vi "Main.vi"() -> ()   [LabVIEW 2016]
uses:
  Spreadsheet filling/Controls/Language Control.ctl
  <vilib>/Platform/TimedLoop/XDataNode/timing_clust.ctl
  <vilib>/Platform/TimedLoop/XDataNode/nitl_modes.ctl
  <vilib>/Platform/TimedLoop/XDataNode/wakeup.ctl
  types/final data type.ctl
  <vilib>/Utility/config.llb/Read Key (Boolean).vi
  <vilib>/Platform/TimedLoop/XDataNode/XDataNode.xnode
  <vilib>/Platform/TimedLoop/XDataNode/XDNodeRunTimeDep.lvlib
  <vilib>/Utility/config.llb/NI_LVConfig.lvlib
panel:
  in  "Gas":bool
  out "Volume % Difference":dbl
  out "Progress":dbl(slide) scale=0.0..100.0
  in  "Software Version":string="1.09(US)"
  out "Sample in progress":bool
  out "Collect info done":bool
  in  "Sample method 2":u16(ring) items=["None", "Pulse Input", "Current Input", "Serial Input"]
  out "Mass % Difference":dbl
  in  "Sample \ninterval (S)":dbl=30.0
  in  "Language":T1
  in  "Collect info":bool
  in  "Export report":bool
  in  "Reset table":bool
  in  "Setpoint \n(kg/min)":dbl
  out "Data table":string[][](table)
  in  "Sample method 1":u16(ring) items=["None", "Pulse Input", "Current Input", "Serial Input"]
  in  "Begin pulse sample":bool
  in  "Transfer Data":bool
  in  "Run #":u16
  # "Mass\n(UUT)"
  # "Mass\n(Master)"
  # "Mass \n% diff"
  # "Volume\n(UUT)"
  # "Volume\n(Master)"
  # "Setpoint"
  # "Run"
  # "Select an input type"
  # "Select an input type"
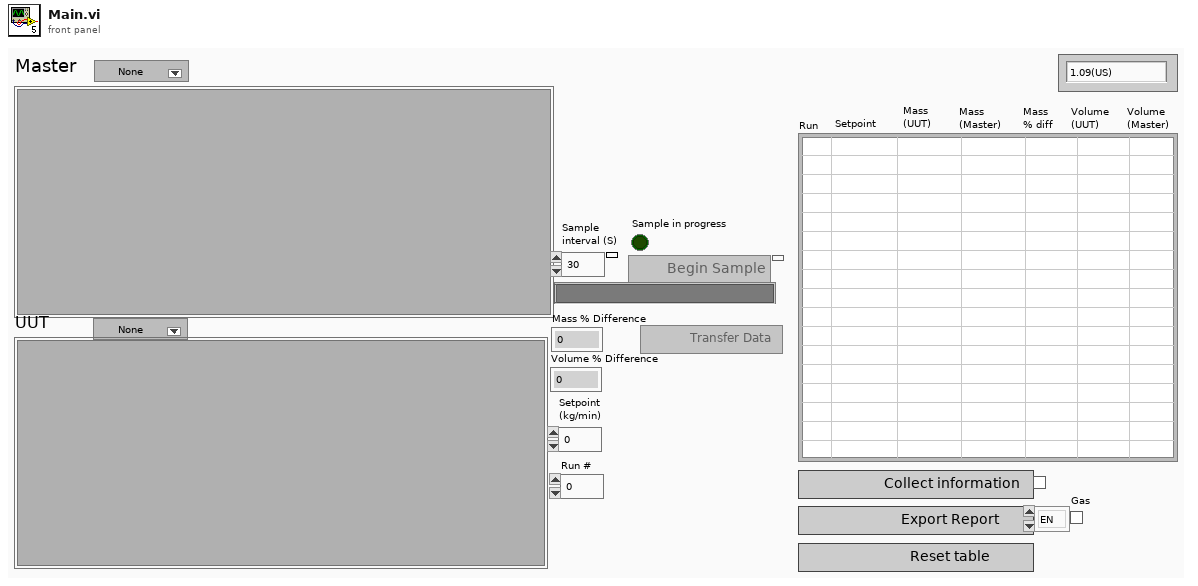
[diagram p1: front panel]
types:
  T1 = typedef "Language Control.ctl" = enum16{"EN", "ES", "FR", "RU"}
  T2 = typedef "final data type.ctl" = cluster{"Master final data":cluster{"Mass total":dbl, "Volume total":dbl, "Density mean":dbl}, "UUT final data":cluster{"Mass total":dbl, "Volume total":dbl, "Density mean":dbl}}
  T3 = enum16{"Init", "Transfer data", "Sample started", "Sample complete"}
  T4 = typedef "XDNodeRunTimeDep.lvlib/timing_clust.ctl" = cluster{"Expected End [f-1]":u64, "Actual End [f-1]":u64, "Finished Late? [f-1]":bool, "Expected End [i-1]":u64, "Actual End [i-1]":u64, "Finished Late? [i-1]":bool, "Expected Start [i]":u64, "Actual Start [i]":u64, "Expected Start [f]":u64, "Actual Start [f]":u64, "Source Name":string, "Structure Name":string, "Period":i64, "Deadline":i64, "Offset":i64, "Start":i64, "Priority":i32, "Timeout":i32, "Mode":T5, "Wakeup Reason":T6, "Error":errorcluster, "Source Type":string, "Secondary Source Type":string, "Global End Time":u64, "Global Start Time":u64, "Frame Duration":u64, "Iteration Duration":u64, "Assigned CPU":i32, "I/O Scan Engine Mode":u32}
  T5 = typedef "XDNodeRunTimeDep.lvlib/nitl_modes.ctl" = enum32{"No Change", "Process missed periods, maintain original phase", "Discard missed periods, maintain original phase", "Process missed periods, ignore original phase", "Discard missed periods, ignore original phase"}
  T6 = typedef "XDNodeRunTimeDep.lvlib/wakeup.ctl" = enum32{"Normal", "Aborted", "Asynchronous wakeup", "Timing source error", "Timed loop error", "Timeout"}
  T7 = enum8{"Enabled", "Disabled", "Disabled and Grayed Out"}
  T8 = typedef "NI_LVConfig.lvlib/Config Data RefNum.ctl" = refnum<k1>
  T9 = typedef "Information_tab_type.ctl" = cluster{"Test Date and Time, 1":string, "Test Comments,3":string, "Sensor Serial Number,6":string, "Sensor Model,7":string, "Size,8":string, "Material,9":string, "Press rating, 10":string, "Temp rating, 11":string, "FCF, 14":string, "D1, 15":string, "D2, 16":string, "K1, 17":string, "K2, 18":string, "FD, 19":string, "Density Temp Coeff, 20":string, "Transmitter Serial Number,23":string, "Transmitter Model Number,24":string, "Mass Flow Units, 25":string, "Density Units, 26":string, "Temperature Units, 27":string, "Mass Flow Cutoff, 28":string, "Mass Flow Damping, 29":string, "Flow Direction, 30":string, "Frequency Flow Rate, 31":string, "Frequency Span, 32":string, "Flow Accuracy, 35":string, "Flow Repeatability, 36":string, "Zero Stability, 37":string, "Density Accuracy, 38":string, "Density Repeatability, 39":string, "Nomincal Flow Rate, 41":string, "Meter Zero, 43":string, "Status, 45":string, "Customer name, 46":string, "Customer address, 47":string, "Sales order number, 48":string, "Technician Name, 49":string, "ref meter, 50":string, "product code,51":string, "fluid,52":string, "fluid temp,53":string}
  T10 = enum16{"0-1-2-3", "2-3-0-1", "1-0-3-2", "3-2-1-0"}
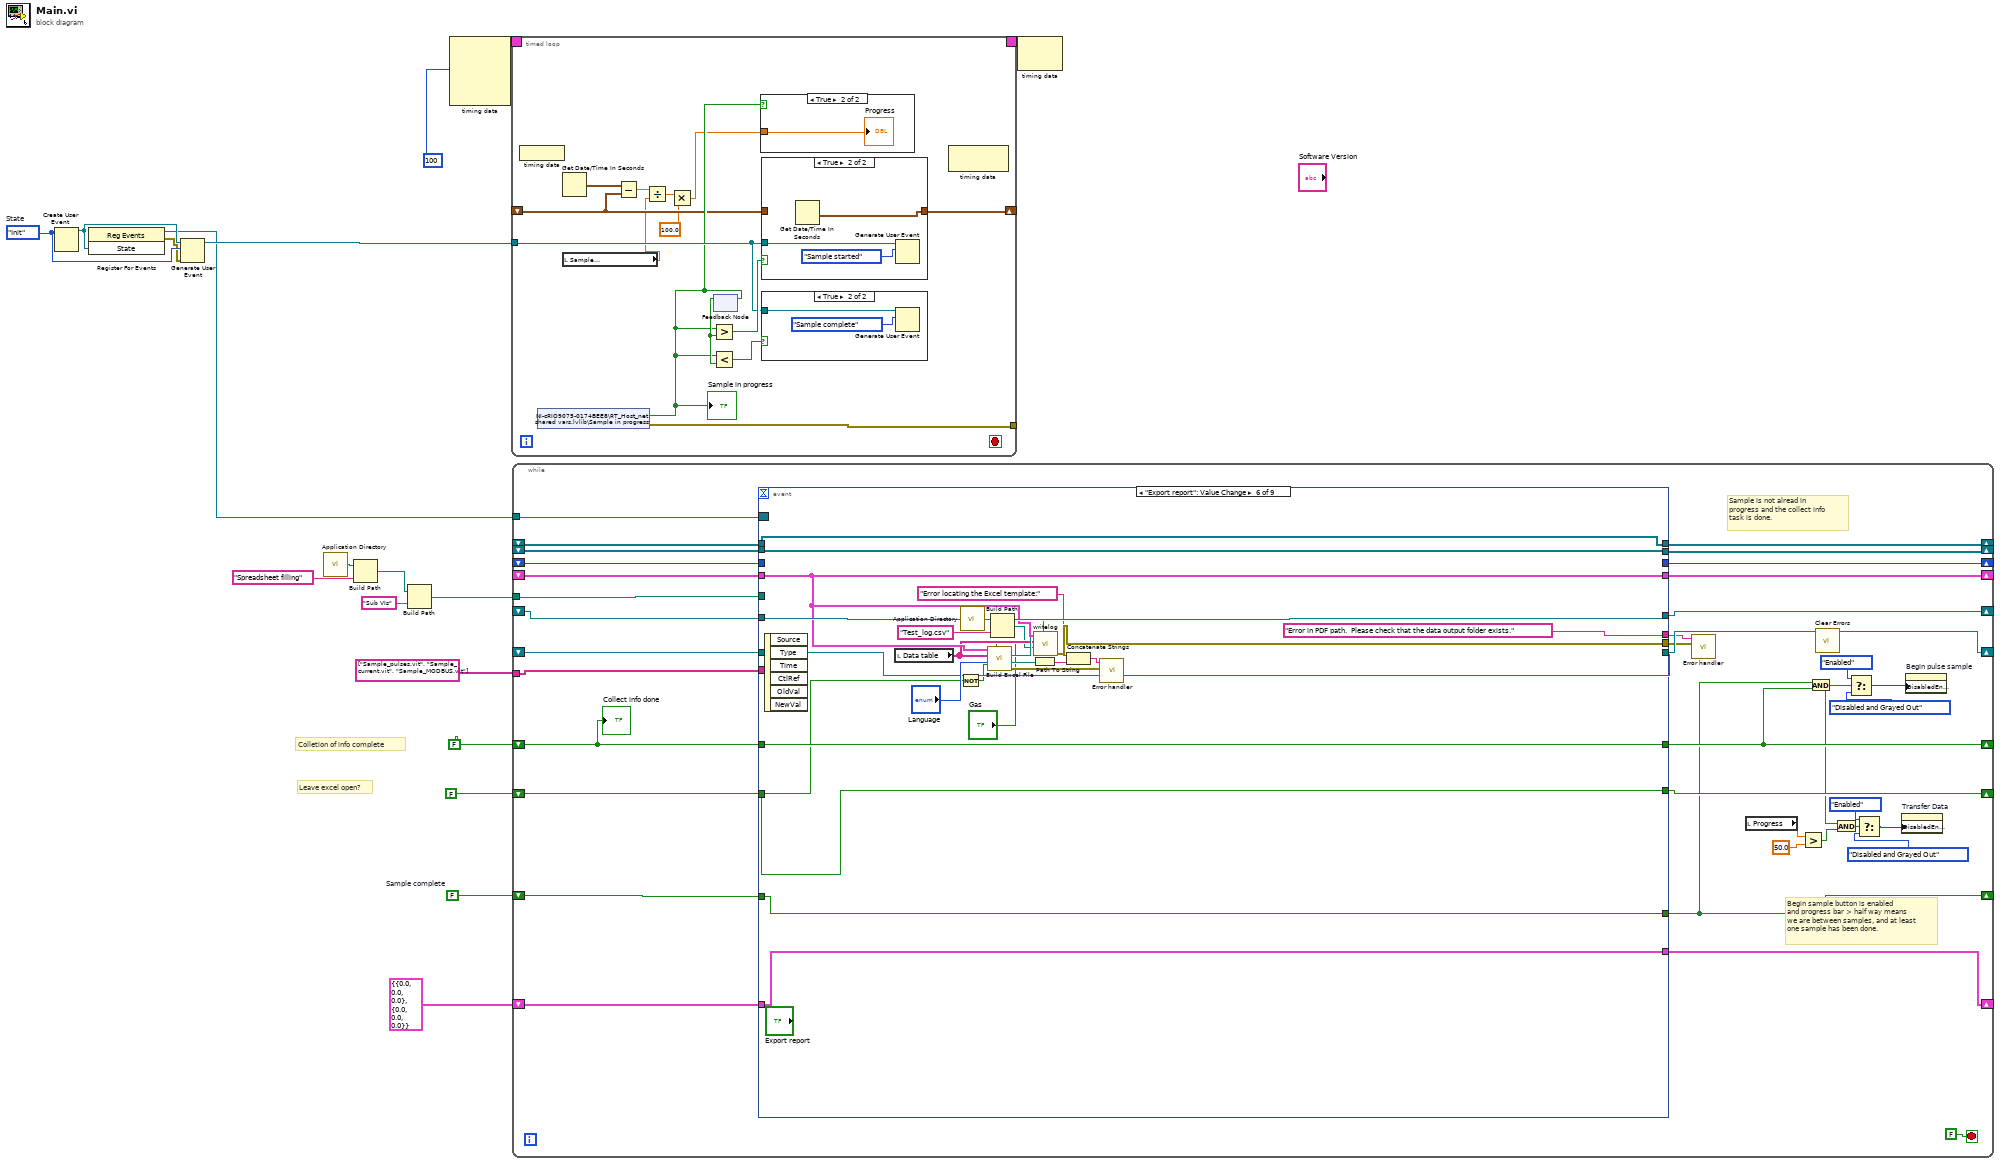
[diagram p0: block diagram]
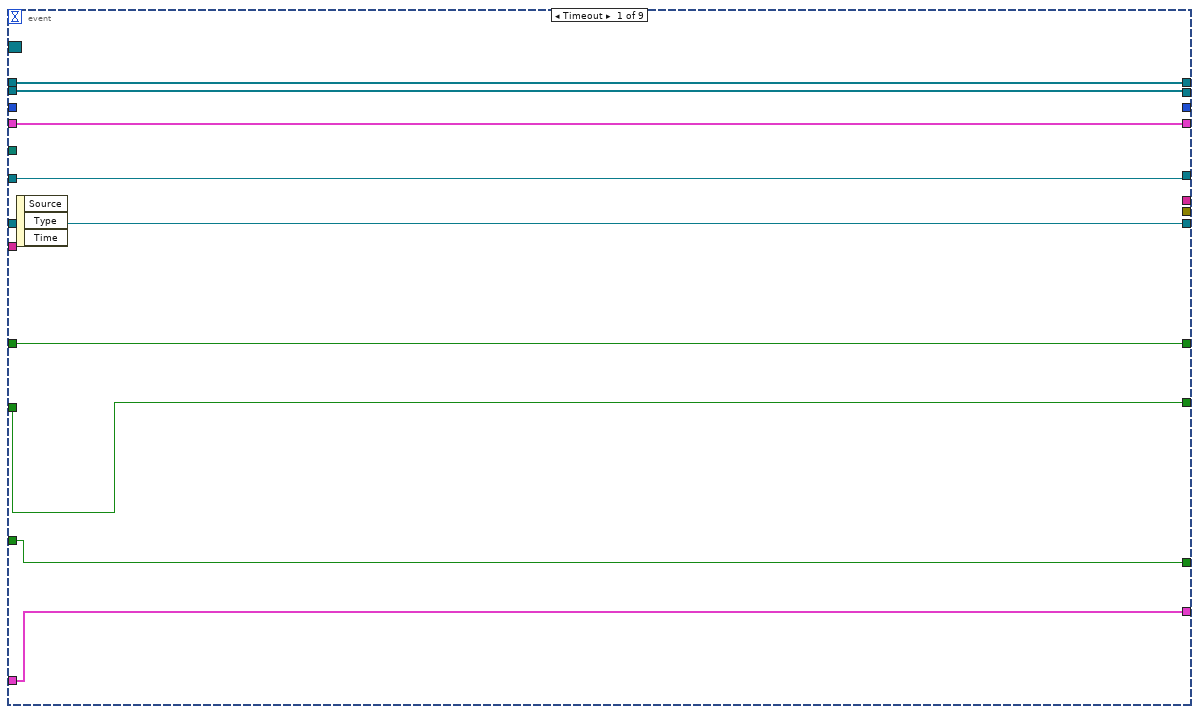
[diagram p5: hidden frame]
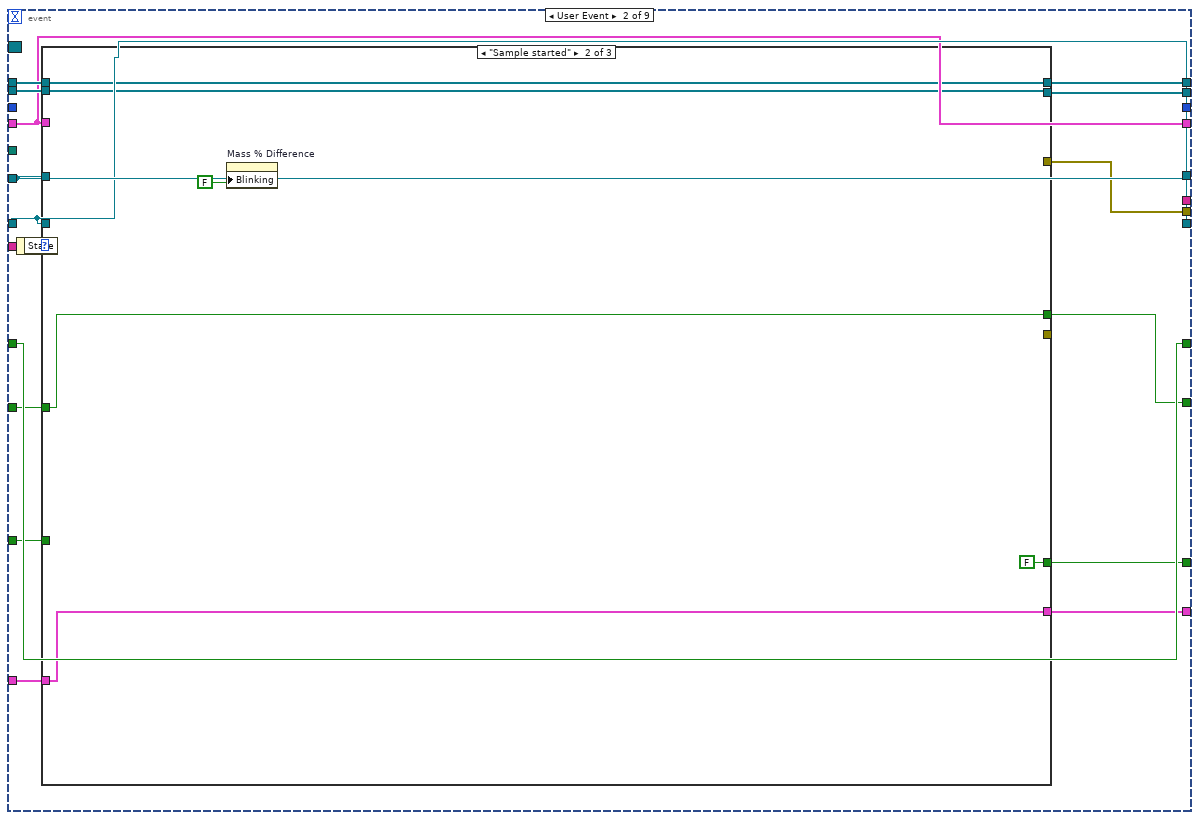
[diagram p6: hidden frame]
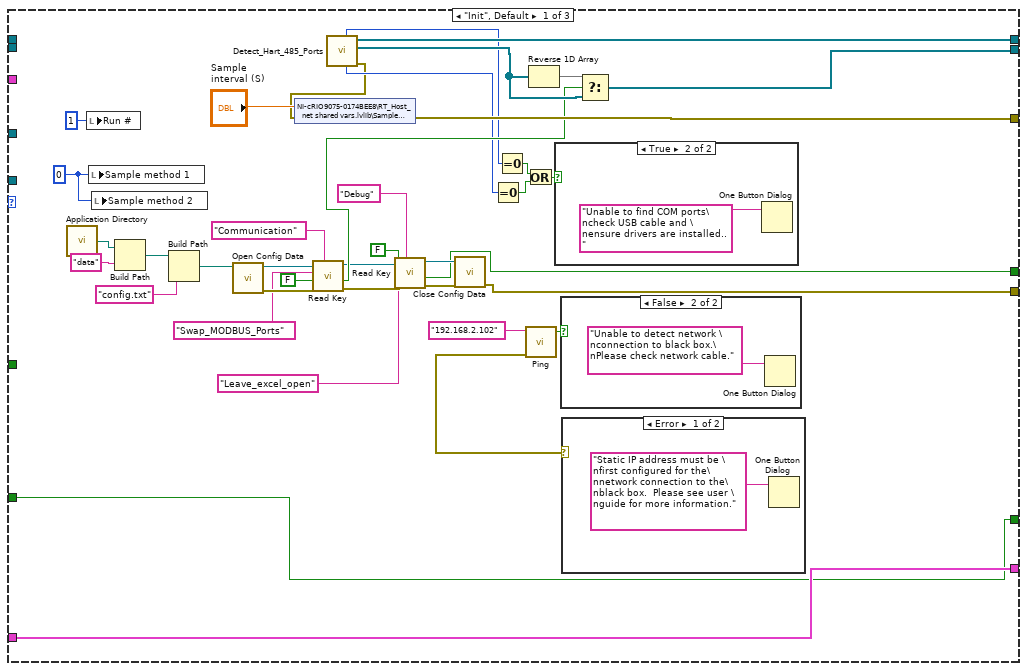
[diagram p7: hidden frame]
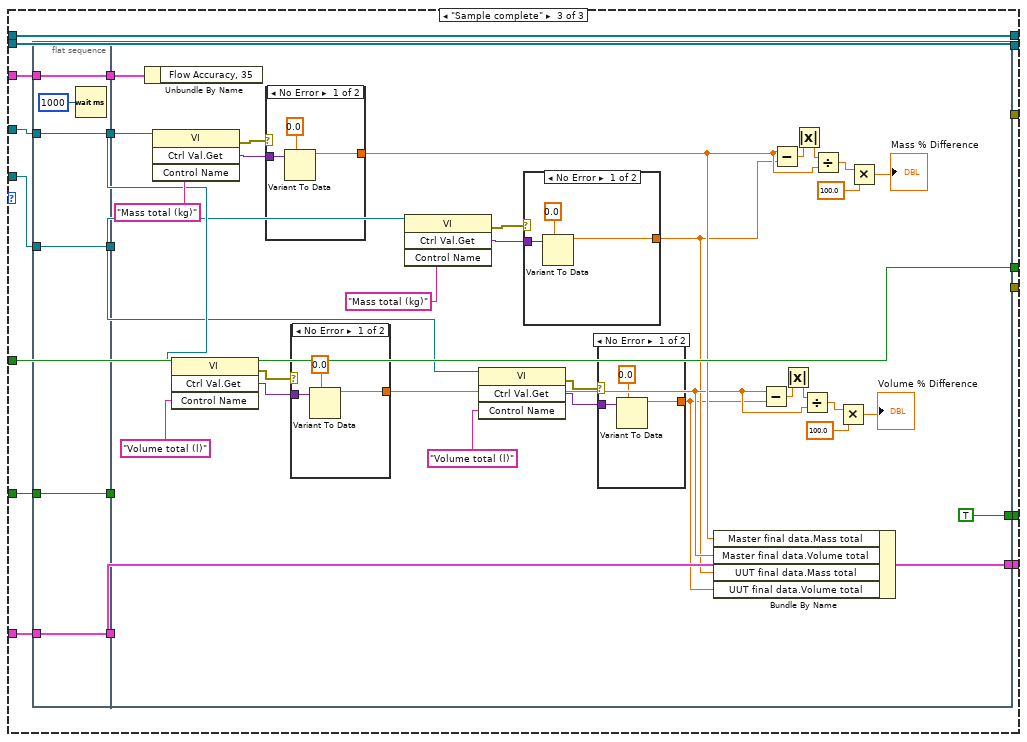
[diagram p11: hidden frame]
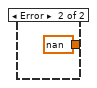
[diagram p12: hidden frame]
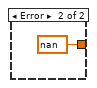
[diagram p13: hidden frame]
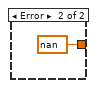
[diagram p14: hidden frame]
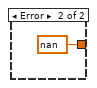
[diagram p15: hidden frame]
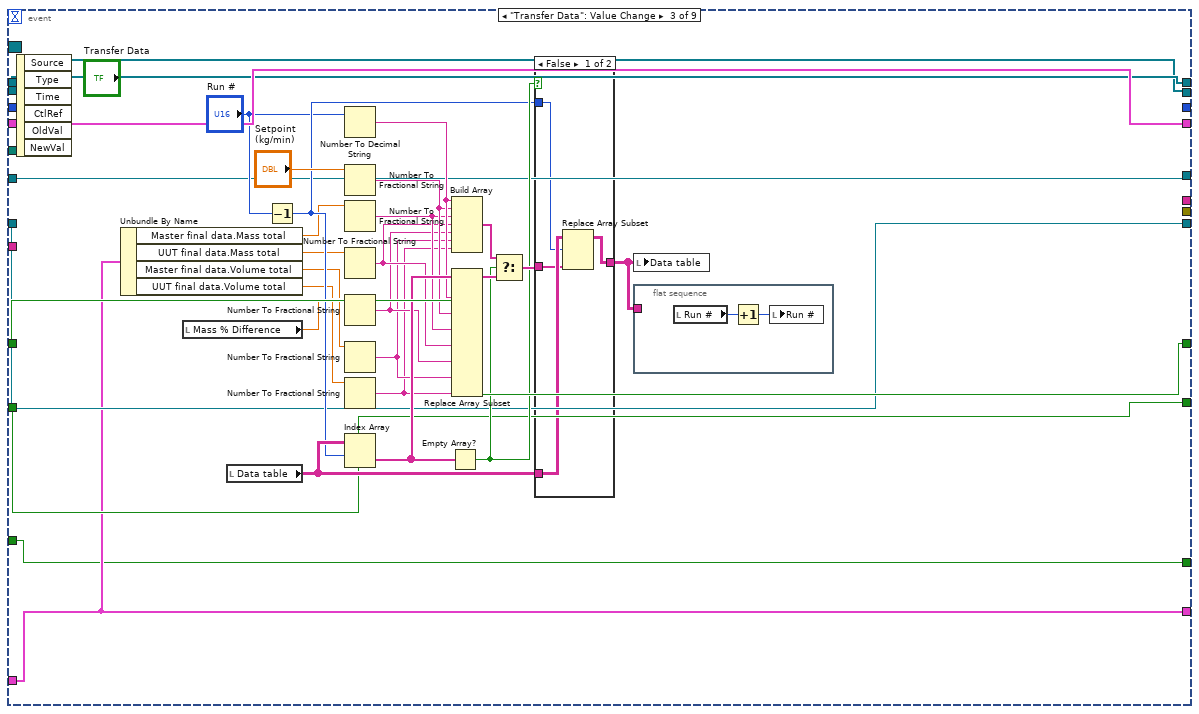
[diagram p16: hidden frame]
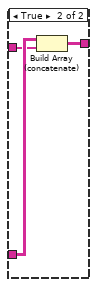
[diagram p17: hidden frame]
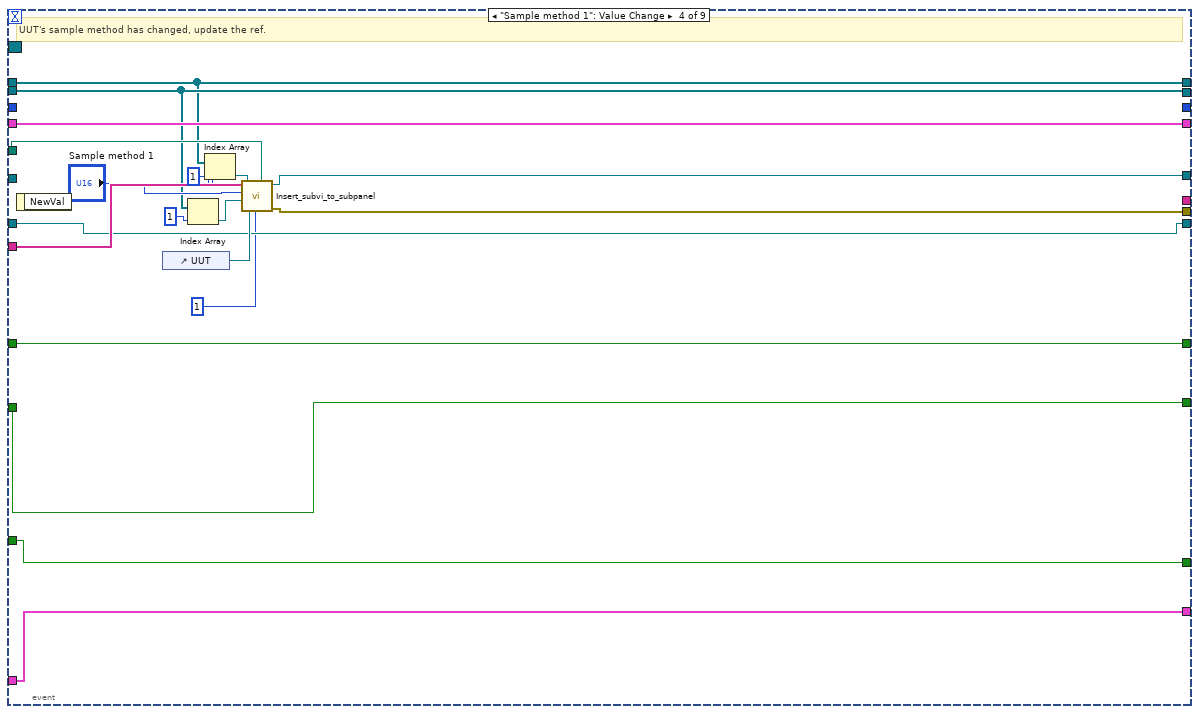
[diagram p18: hidden frame]
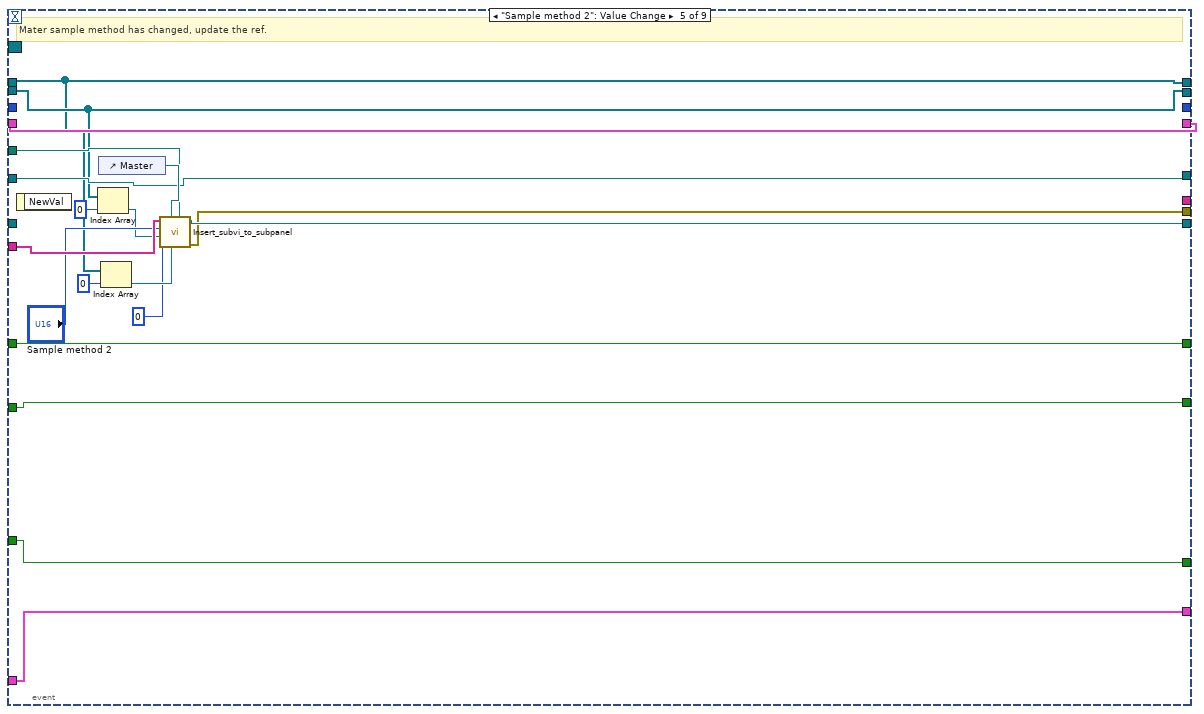
[diagram p19: hidden frame]
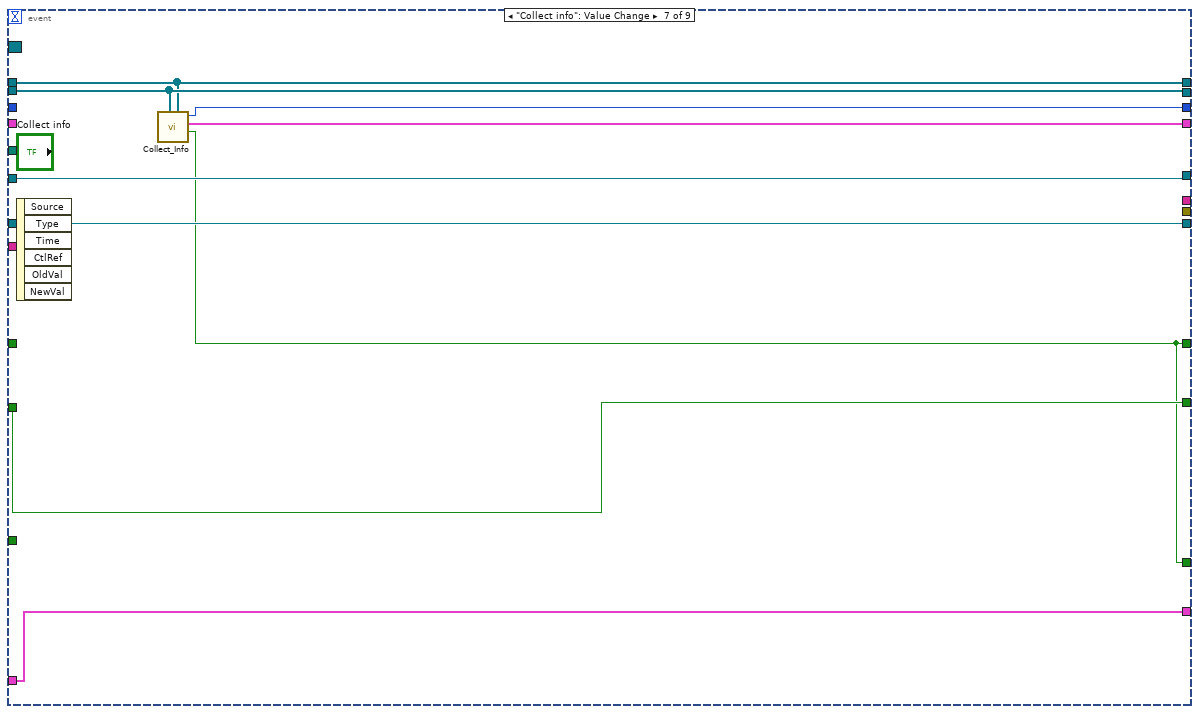
[diagram p20: hidden frame]
diagram:
  w1 = FALSE  # Sample complete
  w12 = T3."Init"  # State
  # "Leave excel open?"
  # "Colletion of info complete"
  n1 = Create User Event(user event datatype=w12) -> (user event=w11:refnum<user-event>)  [unwired: 1 in, 1 out]
  n2 = register-events(w11) -> (reference out=w4:refnum<event-registration>, error out=w10:errorcluster)  [unwired: 2 in]
  n3 = Generate User Event(user event=w11, event data cluster=w12, error in=w10) -> (user event out=w5:refnum<user-event>)  [unwired: 1 in, 1 out]
  n4 = call <vilib>:"Application Directory.vi"() -> ("Application Directory"=w18:path)
  n5 = Build Path(base path=w18, name or relative path="Spreadsheet filling") -> (appended path=w16:path)
  n6 = Build Path(base path=w16, name or relative path="Sub VIs") -> (appended path=w14:path)
  n7 = node-c288(i64 100 ("Period")) -> (w8:T4)  [unwired: 3 in]
  n8 = timed-loop {
    timing: w8 -> [_]
    timing-out: [_] -> w7
    tunnel: [w32] -> _
    tunnel: w5 -> [w29]
    shift-right: [w26] -> _
    shift-left: _ -> [w24]
    stop <- _ stop-if-true
    n9 = node-c288() -> ()  [unwired: 1 in]
    n10 = shared-variable "NI-cRIO9075-0174BEE8\\RT_Host_net shared vars.lvlib\\Sample in progress"() -> (w27:bool, error out=w32:errorcluster)  [unwired: 1 in]
    "Sample in progress" <- w27
    n11 = local read "Sample \ninterval (S)"() -> (w22:dbl)
    n12 = Get Date/Time In Seconds() -> (seconds since 1Jan1904=w25:timestamp)
    n13 = Subtract(x=w25, y=w24) -> (x-y=w23:dbl)
    n14 = Divide(x=w23, y=w22) -> (x/y=w21:dbl)
    n15 = Multiply(x=w21, y=100.0) -> (x*y=w19:dbl)
    n16 = feedback-in #1(w27) -> ()
    n17 = feedback #1() -> (w30:bool)  [unwired: 1 in]
    n18 = Greater?(x=w27, y=w30) -> (0:w31:bool)
    n19 = Less?(x=w27, y=w30) -> (x < y?=w28:bool)
    n20 = case shown="True" w27 {
      tunnel: w19 -> [_ w33]
      frame False {
      }
      frame True {
        "Progress" <- w33
      }
    }
    n21 = case shown="True" w31 {
      tunnel: w29 -> [_ w39]
      tunnel: [w36 w37] -> w26
      tunnel: w24 -> [w36 _]
      frame False {
      }
      frame True {
        n22 = Get Date/Time In Seconds() -> (seconds since 1Jan1904=w37:timestamp)
        n23 = Generate User Event(user event=w39, event data cluster=T3."Sample started" ("event data")) -> ()  [unwired: 2 in, 2 out]
      }
    }
    n24 = case shown="True" w28 {
      tunnel: w29 -> [_ w35]
      frame False {
      }
      frame True {
        n25 = Generate User Event(user event=w35, event data cluster=T3."Sample complete" ("event data")) -> ()  [unwired: 2 in, 2 out]
      }
    }
    n26 = node-c288() -> ()  [unwired: 1 in, 1 out]
  }
  n27 = while {
    shift-right: [w77] -> _
    shift-left: _ -> [w74]
    tunnel: string[] ["Sample_pulses.vit", "Sample_current.vit", "Sample_MODBUS.vit"] -> [w76]
    tunnel: w14 -> [w75]
    shift-right: [w73] -> _
    shift-left: _ -> [w72]
    tunnel: w4 -> [w71]
    shift-right: [w45] -> _
    shift-left: FALSE ("Collect info done") -> [w70]
    shift-right: [w69] -> _
    shift-left: _ -> [w68]
    shift-right: [w64] -> _
    shift-left: _ -> [w62]
    shift-right: [w63] -> _
    shift-left: _ -> [w61]
    shift-right: [w59] -> _
    shift-left: FALSE ("Collect info done") -> [w60]
    shift-right: [w56] -> _
    shift-left: _ -> [w55]
    shift-right: [w53] -> _
    shift-left: T2 {"Master final data"={"Mass total"=0.0, "Volume total"=0.0, "Density mean"=0.0}, "UUT final data"={"Mass total"=0.0, "Volume total"=0.0, "Density mean"=0.0}} ("Final data") -> [w54]
    shift-right: [w42] -> _
    shift-left: w1 -> [w43]
    stop <- FALSE stop-if-true
    # "Sample is not alread in\nprogress and the collect info \ntask is done."
    # "Begin sample button is enabled\nand progress bar > half way means \nwe are between samples, and at least\none sample has been done."
    n28 = event shown="[5] \"Export report\": Value Change" {
      selector: w71 -> [_ _ _ _ _ _ _ _ _]
      dyn-events: _ -> [_ _ _ _ _ _ _ _ _]
      timeout: _ -> [_ _ _ _ _ _ _ _ _]
      tunnel: w76 -> [_ _ _ w279 w296 _ _ _ _]
      tunnel: w75 -> [_ _ _ w271 w290 _ _ _ _]
      tunnel: [w87 w102 w227 w274 w293 w322 w331 w343 w356] -> w77
      tunnel: w74 -> [w87 w102 w227 _ w293 w322 w331 w343 w356]
      tunnel: [w86 w92 w251 w275 w292 w315 w330 w342 w355] -> w73
      tunnel: w72 -> [w86 w92 w251 w275 w292 w315 _ w342 w355]
      tunnel: w70 -> [w85 w101 w250 w272 w298 w320 _ _ w354]
      tunnel: [w85 w101 w250 w272 w298 w320 w323 w341 w354] -> w45
      tunnel: [_ w100 _ w276 w291 w316 _ _ _] -> w58
      tunnel: [w84 w99 w228 w273 w294 w319 w329 w340 w353] -> w69
      tunnel: w68 -> [w84 w99 w228 w273 _ w319 w329 w340 w353]
      tunnel: [w83 w98 w239 w267 w287 w318 w327 w339 w352] -> w64
      tunnel: [w82 w97 w238 w269 w289 w317 w328 w338 w351] -> w63
      tunnel: w62 -> [w83 w96 w239 w267 w287 w318 w327 w339 w352]
      tunnel: w61 -> [w82 w95 w238 w269 w289 w317 w328 w338 w351]
      tunnel: [w81 w94 w233 w263 w284 w309 w326 w333 w350] -> w59
      tunnel: w60 -> [w81 w93 w233 w263 w284 w309 w326 w333 w350]
      tunnel: [_ _ _ _ _ "Error in PDF path.  Please check that the data output folder exists." ("Error reason") _ _ _] -> w57
      tunnel: [_ _ _ _ _ _ w325 _ _] -> w56
      tunnel: w55 -> [_ _ _ _ _ _ _ _ _]
      tunnel: w54 -> [w80 w91 w222 w262 w281 w301 w324 w337 w349]
      tunnel: [w80 w90 w222 w262 w281 w301 w324 w337 w349] -> w53
      tunnel: w43 -> [w79 w89 w221 w261 w280 w300 _ w332 w348]
      tunnel: [w79 w88 w221 w261 w280 w300 w323 w332 w348] -> w42
      event Timeout {
        n29 = event-data() -> ()  [unwired: 1 in, 3 out]
      }
      event User Event {
        n30 = event-data() -> ("State"=w103:T3)  [unwired: 1 in]
        n31 = case shown="\"Sample started\"" w103 {
          tunnel: w102 -> [_ _ w166]
          tunnel: [w140 _ _] -> w100
          tunnel: w99 -> [_ _ w165]
          tunnel: [w139 w151 w164] -> w98
          tunnel: [w125 w150 w163] -> w97
          tunnel: w96 -> [_ w151 w164]
          tunnel: w95 -> [_ w150 w163]
          tunnel: [w107 _ _] -> _
          tunnel: [w106 w149 w160] -> w94
          tunnel: w93 -> [_ w149 w160]
          tunnel: w92 -> [_ _ w158]
          tunnel: w91 -> [w105 w147 w156]
          tunnel: [w105 w147 w155] -> w90
          tunnel: w89 -> [w104 _ w153]
          tunnel: [w104 FALSE ("Sample complete") w152] -> w88
          frame "Init", Default {
            w142 = u16 0 ("Run")
            n32 = call <vilib>:"Application Directory.vi"() -> ("Application Directory"=w136:path)
            n33 = local write "Run #"(u16 1 ("Run #")) -> ()
            n34 = local write "Sample method 1"(w142) -> ()
            n35 = local write "Sample method 2"(w142) -> ()
            n36 = Build Path(base path=w136, name or relative path="data") -> (appended path=w135:path)
            n37 = Build Path(base path=w135, name or relative path="config.txt") -> (appended path=w138:path)
            n38 = call <vilib>:"Open Config Data.vi"("configuration file path"=w138) -> ("error out"=w132:errorcluster, "refnum"=w133:T8)  [unwired: 8 in, 1 out]
            n39 = call-poly <vilib>:"Read Key.vi"("section"="Communication", "error in (no error)"=w132, "default value"=FALSE, "key"="Swap_MODBUS_Ports", "refnum"=w133) -> ("error out"=w113:errorcluster, "value"=w126:bool, "refnum out"=w114:T8)  [unwired: 3 in, 1 out]
            n40 = call "Detect_Hart_485_Ports.vi"() -> ("error out"=w118:errorcluster, "485 Ports"=w128:refnum<visa-resource-name>[], "HART ports"=w139:refnum<visa-resource-name>[], "# 485 ports found"=w124:i32, "# HART ports found"=w123:i32)  [unwired: 6 in, 1 out]
            n41 = shared-variable "NI-cRIO9075-0174BEE8\\RT_Host_net shared vars.lvlib\\Sample period"("Sample \ninterval (S)", error in=w118) -> (error out=w140:errorcluster)
            n42 = call-poly <vilib>:"Read Key.vi"("section"="Debug", "error in (no error)"=w113, "default value"=FALSE, "key"="Leave_excel_open", "refnum"=w114) -> ("error out"=w112:errorcluster, "value"=w106:bool, "refnum out"=w111:T8)  [unwired: 3 in, 1 out]
            n43 = call <vilib>:"Close Config Data.vi"("error in (no error)"=w112, "refnum"=w111) -> ("error out"=w107:errorcluster)  [unwired: 8 in, 1 out]
            n44 = Equal To 0?(x=w124) -> (x = 0?=w121:bool)
            n45 = Equal To 0?(x=w123) -> (x = 0?=w122:bool)
            n46 = Or(x=w122, y=w121) -> (x .or. y?=w120:bool)
            n47 = call "Ping.vi"("Host IP Address"="192.168.2.102") -> ("error out"=w115:errorcluster, "success"=w116:bool)  [unwired: 8 in, 1 out]
            n48 = Reverse 1D Array(array=w128) -> (reversed array=w127:refnum<visa-resource-name>[])
            n49 = case shown="True" w120 {
              frame False {
              }
              frame True {
                n50 = One Button Dialog(message="Unable to find COM ports\ncheck USB cable and \nensure drivers are installed..") -> ()  [unwired: 1 in, 1 out]
              }
            }
            n51 = case shown="False" w116 {
              frame True {
              }
              frame False {
                n52 = One Button Dialog(message="Unable to detect network \nconnection to black box.\nPlease check network cable.") -> ()  [unwired: 1 in, 1 out]
              }
            }
            n53 = case shown="Error" w115 {
              frame Error {
                n54 = One Button Dialog(message="Static IP address must be \nfirst configured for the\nnetwork connection to the\nblack box.  Please see user \nguide for more information.") -> ()  [unwired: 1 in, 1 out]
              }
              frame No Error {
              }
            }
            n55 = Select(t=w127, s=w126, f=w128) -> (s? t:f=w125:refnum<visa-resource-name>[])
          }
          frame "Sample started" {
            n56 = property on="Mass % Difference" class="DigNum (strict)"("Blinking"=FALSE) -> ()  [unwired: 2 in, 2 out]
          }
          frame "Sample complete" {
            n57 = flat-sequence {
              tunnel: w165 -> [w171]
              tunnel: w166 -> [w172]
              tunnel: [w172] -> w162
              tunnel: [w171] -> w161
              tunnel: [w169] -> w159
              tunnel: w158 -> [w169]
              tunnel: [w168] -> w157
              tunnel: w156 -> [w168]
              tunnel: [w167] -> w154
              tunnel: w153 -> [w167]
              tunnel: w162 -> [w191]
              tunnel: w161 -> [w185]
              tunnel: w159 -> [w194]
              tunnel: w157 -> [w179]
              tunnel: [w178] -> w155
              tunnel: w154 -> [_]
              tunnel: [TRUE ("Sample complete")] -> w152
              frame #0 {
                n58 = Wait (ms)(milliseconds to wait=u32 1000) -> ()  [unwired: 1 out]
              }
              frame #1 {
                n59 = Unbundle By Name(w194) -> ()  [unwired: 1 out]
                n60 = invoke class="VI" method="Ctrl Val.Get"(reference=w191, "Control Name"="Mass total (kg)") -> (error out=w204:errorcluster, "Get Control Value Variant"=w203:variant)  [unwired: 2 in, 2 out]
                n61 = invoke class="VI" method="Ctrl Val.Get"(reference=w191, "Control Name"="Volume total (l)") -> (error out=w190:errorcluster, "Get Control Value Variant"=w189:variant)  [unwired: 2 in, 2 out]
                n62 = case shown="No Error" w204 {
                  tunnel: w203 -> [w215 _]
                  tunnel: [w213 nan ("Mass total")] -> w177
                  frame No Error {
                    n63 = Variant To Data(type=0.0 ("Mass total"), Variant=w215) -> (data=w213:dbl)  [unwired: 1 in, 1 out]
                  }
                  frame Error {
                  }
                }
                n64 = case shown="No Error" w190 {
                  tunnel: w189 -> [w211 _]
                  tunnel: [w209 nan ("Mass total")] -> w176
                  frame No Error {
                    n65 = Variant To Data(type=0.0 ("Mass total"), Variant=w211) -> (data=w209:dbl)  [unwired: 1 in, 1 out]
                  }
                  frame Error {
                  }
                }
                n66 = invoke class="VI" method="Ctrl Val.Get"(reference=w185, "Control Name"="Mass total (kg)") -> (error out=w201:errorcluster, "Get Control Value Variant"=w200:variant)  [unwired: 2 in, 2 out]
                n67 = invoke class="VI" method="Ctrl Val.Get"(reference=w185, "Control Name"="Volume total (l)") -> (error out=w187:errorcluster, "Get Control Value Variant"=w188:variant)  [unwired: 2 in, 2 out]
                n68 = case shown="No Error" w201 {
                  tunnel: w200 -> [w219 _]
                  tunnel: [w217 nan ("Mass total")] -> w175
                  frame No Error {
                    n69 = Variant To Data(type=0.0 ("Mass total"), Variant=w219) -> (data=w217:dbl)  [unwired: 1 in, 1 out]
                  }
                  frame Error {
                  }
                }
                n70 = case shown="No Error" w187 {
                  tunnel: w188 -> [w207 _]
                  tunnel: [w205 nan ("Mass total")] -> w174
                  frame No Error {
                    n71 = Variant To Data(type=0.0 ("Mass total"), Variant=w207) -> (data=w205:dbl)  [unwired: 1 in, 1 out]
                  }
                  frame Error {
                  }
                }
                n72 = Bundle By Name(cluster=w179, "Master final data.Mass total"=w177, "Master final data.Volume total"=w176, "UUT final data.Mass total"=w175, "UUT final data.Volume total"=w174) -> (w178:T2)
                n73 = Subtract(x=w176, y=w174) -> (x-y=w183:dbl)
                n74 = Subtract(x=w177, y=w175) -> (x-y=w196:dbl)
                n75 = Absolute Value(x=w183) -> (abs(x)=w184:dbl)
                n76 = Absolute Value(x=w196) -> (abs(x)=w195:dbl)
                n77 = Divide(x=w184, y=w176) -> (x/y=w181:dbl)
                n78 = Divide(x=w195, y=w177) -> (x/y=w198:dbl)
                n79 = Multiply(x=w181, y=100.0) -> (x*y=→"Volume % Difference":dbl)
                n80 = Multiply(x=w198, y=100.0) -> (x*y=→"Mass % Difference":dbl)
              }
            }
          }
        }
      }
      event "Transfer Data": Value Change {
        n81 = event-data() -> ()  [unwired: 1 in, 6 out]
        n82 = Unbundle By Name(w222) -> ("Master final data.Mass total"=w226:dbl, "UUT final data.Mass total"=w225:dbl, "Master final data.Volume total"=w224:dbl, "UUT final data.Volume total"=w223:dbl)
        n83 = local read "Mass % Difference"() -> (w232:dbl)
        n84 = local read "Data table"() -> (w241:string[][])
        n85 = Decrement(x="Run #") -> (x-1=w237:u16)
        n86 = Number To Decimal String(number="Run #") -> (decimal integer string=w247:string)  [unwired: 1 in]
        n87 = Number To Fractional String(number="Setpoint \n(kg/min)") -> (F-format string=w246:string)  [unwired: 3 in]
        n88 = Number To Fractional String(number=w226) -> (F-format string=w245:string)  [unwired: 3 in]
        n89 = Number To Fractional String(number=w225) -> (F-format string=w234:string)  [unwired: 3 in]
        n90 = Number To Fractional String(number=w232) -> (F-format string=w231:string)  [unwired: 3 in]
        n91 = Number To Fractional String(number=w224) -> (F-format string=w230:string)  [unwired: 3 in]
        n92 = Number To Fractional String(number=w223) -> (F-format string=w229:string)  [unwired: 3 in]
        n93 = Index Array(array=w241, index (row)=w237) -> (element=w248:string[])  [unwired: 1 in]
        n94 = Empty Array?(array=w248) -> (empty?=w240:bool)
        n95 = Build Array(w247, w246, w245, w234, w231, w230, w229) -> (w243:string[])
        n96 = Replace Array Subset(array=w248, new element #1=w247, new element #2=w246, new element #3=w245, new element #4=w234, new element #5=w231, new element #6=w230, new element #7=w229) -> (w244:string[])  [unwired: 7 in]
        n97 = Select(t=w243, s=w240, f=w244) -> (s? t:f=w242:string[])
        n98 = case shown="False" w240 {
          tunnel: w241 -> [w257 w260]
          tunnel: [w256 w259] -> w235
          tunnel: w237 -> [w255 _]
          tunnel: w242 -> [w254 w258]
          frame False {
            n99 = Replace Array Subset(array=w257, new element=w254, index (row)=w255) -> (w256:string[][])  [unwired: 1 in]
          }
          frame True {
            n100 = Build Array (concatenate)(w260, w258) -> (w259:string[][])
          }
        }
        n101 = local write "Data table"(w235) -> ()
        n102 = flat-sequence {
          tunnel: w235 -> [_]
          frame #0 {
            n103 = local read "Run #"() -> (w253:u16)
            n104 = Increment(x=w253) -> (x+1=w252:u16)
            n105 = local write "Run #"(w252) -> ()
          }
        }
      }
      event "Sample method 1": Value Change {
        # "UUT's sample method has changed, update the ref."
        n106 = event-data() -> ()  [unwired: 1 in, 1 out]
        n107 = control-ref of="UUT"() -> (w277:refnum<vi>)
        n108 = Index Array(array=w269, index=1) -> (element=w270:refnum<visa-resource-name>)
        n109 = Index Array(array=w267, index=1) -> (element=w268:refnum<visa-resource-name>)
        n110 = call "Insert_subvi_to_subpanel.vi"("SubVI path"=w271, "HART resource name"=w268, "subpanel ref"=w277, "Input number"=1, "MODBUS resource name"=w270, "Index"="Sample method 1", "Array of VIs to insert"=w279) -> ("error out"=w276:errorcluster, "VI reference out"=w274:refnum<vi>)  [unwired: 3 in]
      }
      event "Sample method 2": Value Change {
        # "Mater sample method has changed, update the ref."
        n111 = event-data() -> ()  [unwired: 1 in, 1 out]
        n112 = Index Array(array=w289, index=0) -> (element=w288:refnum<visa-resource-name>)
        n113 = control-ref of="Master"() -> (w297:refnum<vi>)
        n114 = Index Array(array=w287, index=0) -> (element=w286:refnum<visa-resource-name>)
        n115 = call "Insert_subvi_to_subpanel.vi"("SubVI path"=w290, "HART resource name"=w286, "subpanel ref"=w297, "Input number"=0, "MODBUS resource name"=w288, "Index"="Sample method 2", "Array of VIs to insert"=w296) -> ("error out"=w291:errorcluster, "VI reference out"=w294:refnum<vi>)  [unwired: 3 in]
      }
      event "Export report": Value Change {
        n116 = event-data() -> ()  [unwired: 1 in, 6 out]
        n117 = local read "Data table"() -> (w313:string[][])
        n118 = Not(x=w309) -> (.not. x?=w308:bool)
        n119 = call <vilib>:"Application Directory.vi"() -> ("Application Directory"=w312:path)
        n120 = call "Build Excel File.vi"("close report? (T)"=w308, "Gas"="Gas", "Language"="Language", "Raw data"=w313, "Information"=w315) -> ("error out"=w306:errorcluster, "Excel path"=w304:path, "PDF path out"=w314:path)  [unwired: 3 in, 1 out]
        n121 = Build Path(base path=w312, name or relative path="Test_log.csv") -> (appended path=w310:path)
        n122 = Path To String(path=w304) -> (string=w302:string)
        n123 = call "writelog.vi"("PDF path in"=w314, "data file path"=w310, "Data table"=w313, "Information"=w315) -> ("error out"=w316:errorcluster)  [unwired: 7 in]
        n124 = Concatenate Strings("Error locating the Excel template:" ("Error reason"), w302) -> (w303:string)
        n125 = call "Error handler.vi"("error in"=w306, "Error reason"=w303) -> ()  [unwired: 10 in]
      }
      event "Collect info": Value Change {
        n126 = event-data() -> ()  [unwired: 1 in, 6 out]
        n127 = call "Collect_Info.vi"("HART ports"=w327, "485 Ports"=w328) -> ("Read Completed"=w323:bool, "Information"=w330:T9, "Byte order"=w325:T10)  [unwired: 7 in]
      }
      event "Reset table": Value Change {
        n128 = event-data() -> ()  [unwired: 1 in, 6 out]
        n129 = Two Button Dialog(message="Are you sure?", 2:"Yes" ("T button name (\"OK\")")) -> (T button?=w334:bool)  [unwired: 1 in]
        n130 = case shown="True" w334 {
          tunnel: [w344 FALSE ("Collect info done")] -> w341
          tunnel: w333 -> [w344 _]
          frame False {
          }
          frame True {
            # "Reset table and run counter"
            # "Reset collection info status"
            n131 = local write "Run #"(u16 1 ("Run")) -> ()
            "Data table" <- string[][] [] ("Raw data")
          }
        }
      }
      event "Begin pulse sample": Value Change {
        n132 = event-data() -> ()  [unwired: 1 in, 6 out]
      }
    }
    n133 = call "Error handler.vi"("error in"=w58, "Error reason"=w57) -> ()  [unwired: 10 in]
    n134 = local read "Progress"() -> (w48:dbl)
    n135 = Greater?(x=w48, y=50.0) -> (0:w46:bool)
    n136 = And(x=w42, y=w45) -> (x .and. y?=w44:bool)
    n137 = call <vilib>:"Clear Errors.vi"() -> ()  [unwired: 6 in, 2 out]
    n138 = And(x=w44, y=w46) -> (x .and. y?=w49:bool)
    n139 = Select(t=T7."Enabled" ("Disabled"), s=w44, f=T7."Disabled and Grayed Out" ("Disabled")) -> (s? t:f=w65:T7)
    n140 = Select(t=T7."Enabled" ("Disabled"), s=w49, f=T7."Disabled and Grayed Out" ("Disabled")) -> (s? t:f=w50:T7)
    n141 = property on="Transfer Data" class="Bool"("DisabledEnum"=w50) -> ()  [unwired: 2 in, 2 out]
    n142 = property on="Begin pulse sample" class="Bool (strict)"("DisabledEnum"=w65) -> ()  [unwired: 2 in, 2 out]
    "Collect info done" <- w70
  }
  n143 = node-c288(w7) -> ()  [unwired: 1 out]
